vi "Append Label to Error.vi"(8 "error in":errorcluster, 10 "pre error":errorcluster, 11 "Label":string) -> (0 "error out":errorcluster)   [LabVIEW 2023, in "Label-Driven UI.lvlib"]
uses:
  Label-Driven UI.lvlib
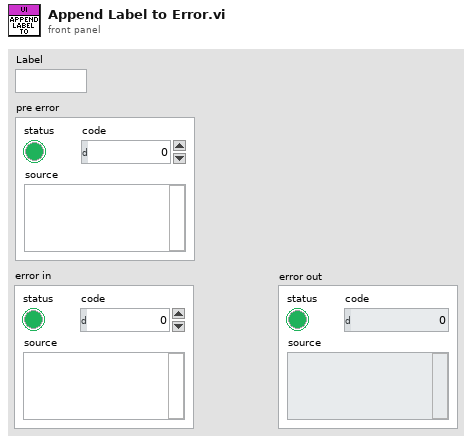
[diagram p1: front panel]
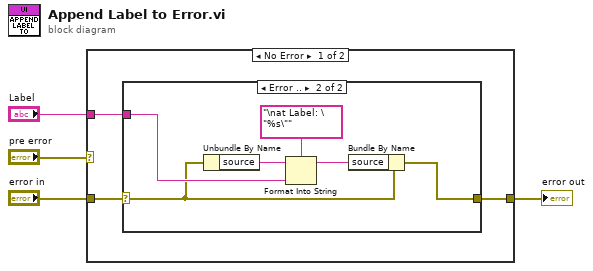
[diagram p0: block diagram]
diagram:
  n1 = case shown="No Error" "pre error" {
    tunnel: "error in" -> [w7 w15]
    tunnel: [w6 w15] -> w2
    tunnel: "Label" -> [w5 _]
    frame No Error {
      n2 = case shown="Error .." w7 {
        selector: w7 -> [w8 w11]
        tunnel: [w8 w10] -> w6
        tunnel: w5 -> [_ w12]
        frame No Error {
        }
        frame Error {
          n3 = Unbundle By Name(w11) -> ("source"=w14:string)
          n4 = Format Into String(format string="\nat Label: \"%s\"", initial string=w14, w12) -> (resulting string=w9:string)  [unwired: 1 in, 1 out]
          n5 = Bundle By Name(cluster=w11, "source"=w9) -> (w10:errorcluster)
        }
      }
    }
    frame Error {
    }
  }
  "error out" <- w2
